vi "Build DashBoard Data.vi"(11 "Dashboard Enables":T3={"Analog Module 1"=[TRUE, TRUE, TRUE, TRUE, TRUE, TRUE, TRUE, TRUE], "Analog Module 2"=[FALSE, FALSE, FALSE, FALSE, FALSE, FALSE, FALSE, FALSE], "Digital Module 1"=TRUE, "Digital Module 2"=FALSE, "Solenoid Module"=TRUE}) -> ()   [LabVIEW 2012]
doc: "This VI builds data and sends it back to the dashboard PC program. By default it sends back the raw values for the first analog, digital, and solenoid module. Modify it to send back the data you want to view. Consider adding higher level data to the Dashboard Datatype.ctl and to this VI. Then update the Dashboard to display the data however you like.\n\nThis software is licensed. Open the labview\\readme\\WPI Robotics Library Open Source License.txt file for more information."
uses:
  DashboardEnable.ctl
  Dashboard Datatype.ctl
  <vilib>/Rock Robotics/WPI/DriverStation/WPI_DriverStationDigitalData.ctl
  Robot Global Data.vi
  <vilib>/Rock Robotics/SystemInterfaces/System/FPGA_SystemGet.vi
panel:
  out "Dashboard Data":T1
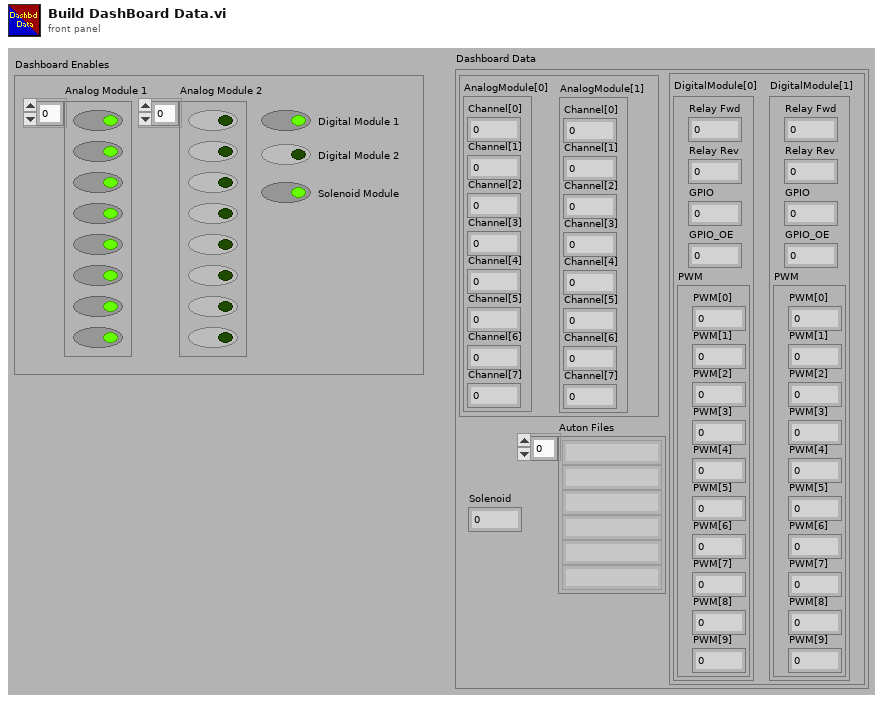
[diagram p1: front panel]
types:
  T1 = typedef "Dashboard Datatype.ctl" = cluster{cluster{"AnalogModule[0]":cluster{"Channel[0]":sgl, "Channel[1]":sgl, "Channel[2]":sgl, "Channel[3]":sgl, "Channel[4]":sgl, "Channel[5]":sgl, "Channel[6]":sgl, "Channel[7]":sgl}, "AnalogModule[1]":cluster{"Channel[0]":sgl, "Channel[1]":sgl, "Channel[2]":sgl, "Channel[3]":sgl, "Channel[4]":sgl, "Channel[5]":sgl, "Channel[6]":sgl, "Channel[7]":sgl}}, cluster{"DigitalModule[0]":T2, "DigitalModule[1]":T2}, "Solenoid":u8, "Auton Files":string[]}
  T2 = typedef "WPI_DriverStationDigitalData.ctl" = cluster{"Relay Fwd":u8, "Relay Rev":u8, "GPIO":u16, "GPIO_OE":u16, "PWM":cluster{"PWM[0]":u8, "PWM[1]":u8, "PWM[2]":u8, "PWM[3]":u8, "PWM[4]":u8, "PWM[5]":u8, "PWM[6]":u8, "PWM[7]":u8, "PWM[8]":u8, "PWM[9]":u8}}
  T3 = typedef "DashboardEnable.ctl" = cluster{"Analog Module 1":bool[], "Analog Module 2":bool[], "Digital Module 1":bool, "Digital Module 2":bool, "Solenoid Module":bool}
  T4 = cluster{"AnalogModule[0]":cluster{"Channel[0]":sgl, "Channel[1]":sgl, "Channel[2]":sgl, "Channel[3]":sgl, "Channel[4]":sgl, "Channel[5]":sgl, "Channel[6]":sgl, "Channel[7]":sgl}, "AnalogModule[1]":cluster{"Channel[0]":sgl, "Channel[1]":sgl, "Channel[2]":sgl, "Channel[3]":sgl, "Channel[4]":sgl, "Channel[5]":sgl, "Channel[6]":sgl, "Channel[7]":sgl}}
  T5 = cluster{"Channel[0]":sgl, "Channel[1]":sgl, "Channel[2]":sgl, "Channel[3]":sgl, "Channel[4]":sgl, "Channel[5]":sgl, "Channel[6]":sgl, "Channel[7]":sgl}[]
  T6 = cluster{"Channel[0]":sgl, "Channel[1]":sgl, "Channel[2]":sgl, "Channel[3]":sgl, "Channel[4]":sgl, "Channel[5]":sgl, "Channel[6]":sgl, "Channel[7]":sgl}
  T7 = cluster{"AnalogModule[0][0]":sgl, "AnalogModule[0][1]":sgl, "AnalogModule[0][2]":sgl, "AnalogModule[0][3]":sgl, "AnalogModule[0][4]":sgl, "AnalogModule[0][5]":sgl, "AnalogModule[0][6]":sgl, "AnalogModule[0][7]":sgl}
  T8 = cluster{"[0]":cluster{"Channel[0]":sgl, "Channel[1]":sgl, "Channel[2]":sgl, "Channel[3]":sgl, "Channel[4]":sgl, "Channel[5]":sgl, "Channel[6]":sgl, "Channel[7]":sgl}, "[1]":cluster{"Channel[0]":sgl, "Channel[1]":sgl, "Channel[2]":sgl, "Channel[3]":sgl, "Channel[4]":sgl, "Channel[5]":sgl, "Channel[6]":sgl, "Channel[7]":sgl}}
  T9 = cluster{"DigitalModule[0]":T2, "DigitalModule[1]":T2}
  T10 = typedef "FPGA_DIODevRef.ctl" = cluster{"DevStatus":errorcluster, "Module":T11}
  T11 = typedef "FPGA_TypedefDigitalModule.ctl" = enum16{"Digital Module 1", "Digital Module 2"}
  T12 = cluster{"[0]":u8, "[1]":u8, "[2]":u8, "[3]":u8, "[4]":u8, "[5]":u8, "[6]":u8, "[7]":u8, "[8]":u8, "[9]":u8}
  T13 = typedef "FPGA_SolenoidDevRef.ctl" = cluster{"DevStatus":errorcluster, "Module":T14}
  T14 = typedef "FPGA_TypedefSolenoidModule.ctl" = enum16{"Solenoid Module 1", "Solenoid Module 2"}
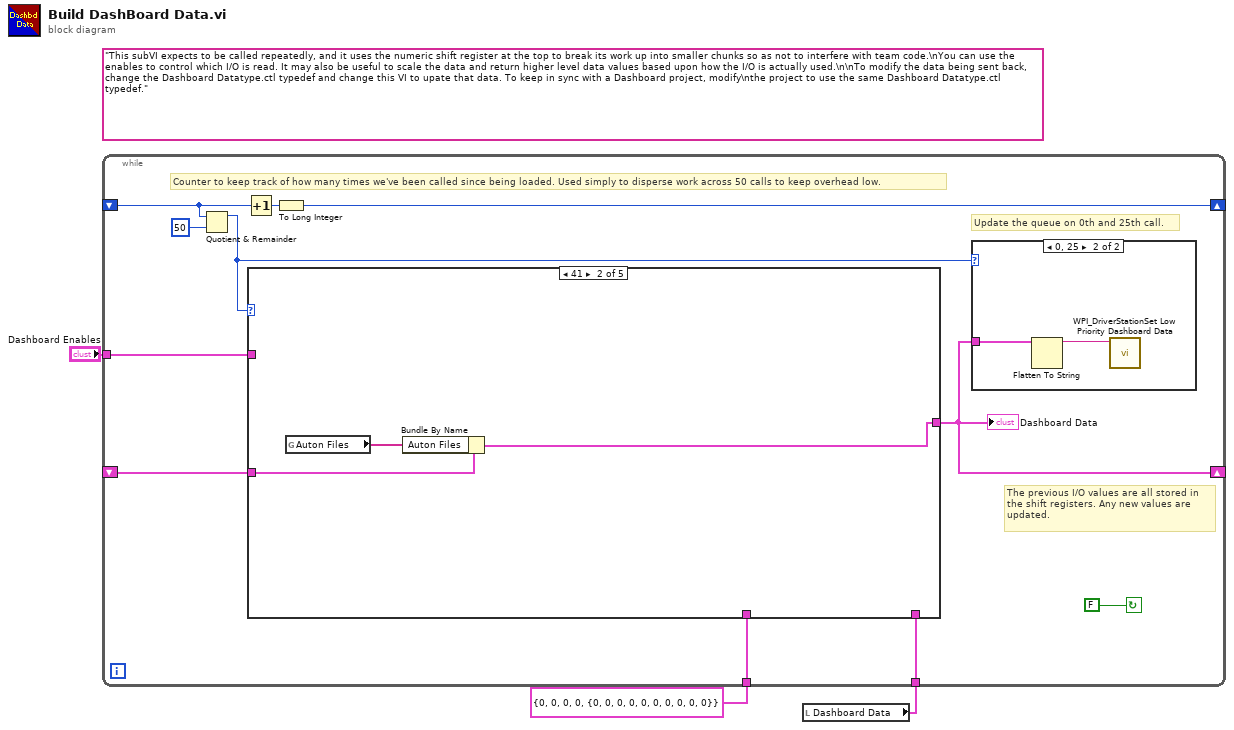
[diagram p0: block diagram]
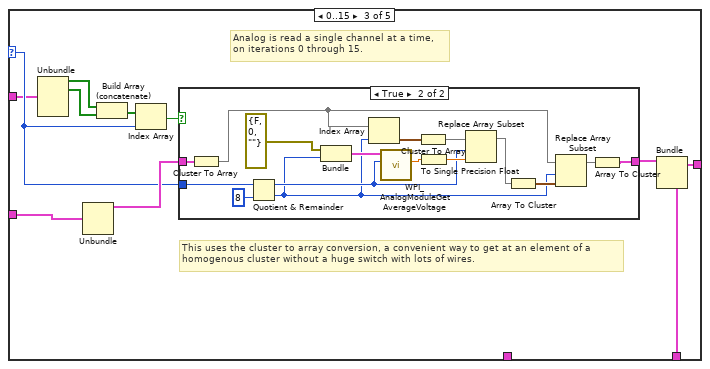
[diagram p4: hidden frame]
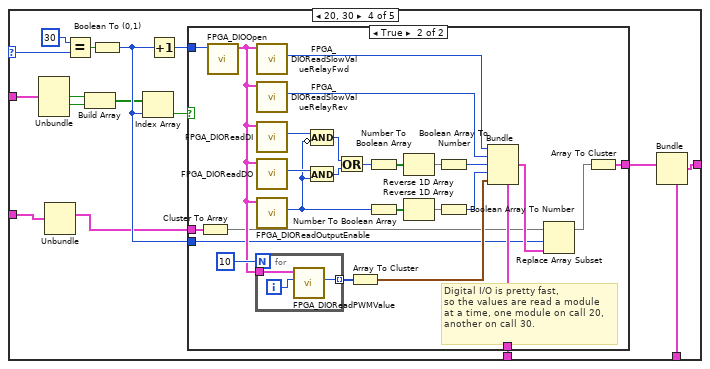
[diagram p6: hidden frame]
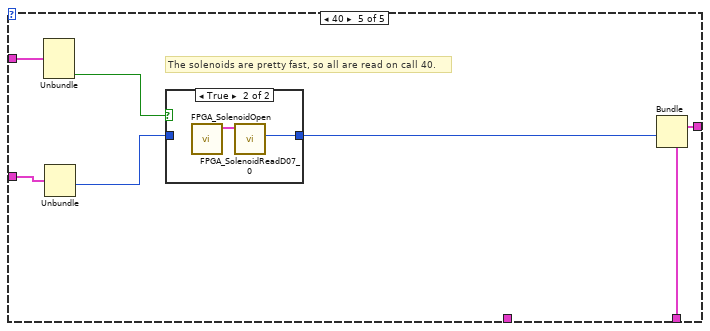
[diagram p8: hidden frame]
diagram:
  (unwired) "This subVI expects to be called repeatedly, and it uses the numeric shift register at the top to break its work up into smaller chunks so as not to interfere with team code.\nYou can use the enables to control which I/O is read. It may also be useful to scale the data and return higher level data values based upon how the I/O is actually used.\n\nTo modify the data being sent back, change the Dashboard Datatype.ctl typedef and change this VI to upate that data. To keep in sync with a Dashboard project, modify\nthe project to use the same Dashboard Datatype.ctl typedef."
  n1 = local read "Dashboard Data"() -> (w2:T1)
  n2 = while {
    shift-right: [w7] -> _
    shift-left: _ -> [w9]
    shift-right: [w4] -> _
    shift-left: _ -> [w12]
    tunnel: T2 {"Relay Fwd"=0, "Relay Rev"=0, "GPIO"=0, "GPIO_OE"=0, "PWM"={"PWM[0]"=0, "PWM[1]"=0, "PWM[2]"=0, "PWM[3]"=0, "PWM[4]"=0, "PWM[5]"=0, "PWM[6]"=0, "PWM[7]"=0, "PWM[8]"=0, "PWM[9]"=0}} ("DigitalModule[1]") -> [w11]
    tunnel: w2 -> [w6]
    tunnel: "Dashboard Enables" -> [w5]
    stop <- FALSE continue-if-true
    # "Counter to keep track of how many times we've been called since being loaded. Used simply to disperse work across 50 calls to keep overhead low."
    # "Update the queue on 0th and 25th call."
    # "The previous I/O values are all stored in\nthe shift registers. Any new values are\nupdated."
    n3 = Quotient & Remainder(x=w9, y=50) -> (x-y*floor(x/y)=w8:i32)  [unwired: 1 out]
    n4 = Increment(x=w9) -> (x+1=w14:i32)
    n5 = case shown="41" w8 {
      selector: w8 -> [_ _ w26 w58 _]
      tunnel: [w17 w19 w22 w49 w98] -> w4
      tunnel: w12 -> [w17 w20 w21 w51 w100]
      tunnel: w11 -> [_ _ _ w64 _]
      tunnel: w6 -> [_ _ w28 w50 w97]
      tunnel: w5 -> [_ _ w25 w56 w101]
      frame Default {
        # "Don't update any I/O"
      }
      frame 41 {
        n6 = global read "Robot Global Data.vi" "Auton Files"() -> (w18:string[])
        n7 = Bundle By Name(cluster=w20, "Auton Files"=w18) -> (w19:T1)
      }
      frame 0..15 {
        # "This uses the cluster to array conversion, a convenient way to get at an element of a\nhomogenous cluster without a huge switch with lots of wires."
        # "Analog is read a single channel at a time,\non iterations 0 through 15."
        n8 = Unbundle(w25) -> ("Analog Module 1"=w24:bool[], "Analog Module 2"=w23:bool[])  [unwired: 3 out]
        n9 = Unbundle(w21) -> (w27:T4)  [unwired: 3 out]
        n10 = Build Array (concatenate)(w24, w23) -> (w30:bool[])
        n11 = Index Array(array=w30, index=w26) -> (element=w31:bool)
        n12 = case shown="True" w31 {
          tunnel: w26 -> [_ w39]
          tunnel: [w32 w36] -> w29
          tunnel: w27 -> [w32 w35]
          frame False {
          }
          frame True {
            n13 = Cluster To Array(cluster=w35) -> (array=w34:T5)
            n14 = Quotient & Remainder(x=w39, y=8) -> (x-y*floor(x/y)=w38:i32, floor(x/y)=w33:i32)
            n15 = Bundle("DevStatus"=errorcluster {"status"=FALSE, "code"=0, "source"=""}, w33) -> (w47:cluster{"DevStatus":errorcluster, i32})  [unwired: 1 out]
            n16 = Index Array(array=w34, index=w33) -> (element=w41:T6)
            n17 = call <vilib>:"WPI_AnalogModuleGetAverageVoltage.vi"("Channel"=w38, "AnalogModuleDevStatus"=w47) -> ("Average Voltage"=w44:dbl)  [unwired: 1 in, 8 out]
            n18 = Cluster To Array(cluster=w41) -> (array=w40:sgl[])
            n19 = To Single Precision Float(number=w44) -> (single precision float=w43:sgl)
            n20 = Replace Array Subset(array=w40, new element=w43, index=w38) -> (w42:sgl[])
            n21 = Array To Cluster(array=w42) -> (cluster=w46:T7)
            n22 = Replace Array Subset(array=w34, new element=w46, index=w33) -> (w37:T5)
            n23 = Array To Cluster(array=w37) -> (cluster=w36:T8)
          }
        }
        n24 = Bundle(cluster=w28, w29) -> (w22:T1)  [unwired: 3 out]
      }
      frame 20, 30 {
        n25 = Unbundle(w56) -> ("Digital Module 1"=w55:bool, "Digital Module 2"=w54:bool)  [unwired: 3 out]
        n26 = Unbundle(w51) -> (w53:T9)  [unwired: 3 out]
        n27 = Equal?(x=30, y=w58) -> (x = y?=w62:bool)
        n28 = Build Array(w55, w54) -> (w57:bool[])
        n29 = Boolean To (0,1)(Boolean=w62) -> (0, 1=w60:i16)
        n30 = Index Array(array=w57, index=w60) -> (element=w59:bool)
        n31 = Increment(x=w60) -> (x+1=w61:i16)
        n32 = case shown="True" w59 {
          tunnel: w64 -> [_ w73]
          tunnel: [w65 w66] -> w52
          tunnel: w61 -> [_ w71]
          tunnel: w60 -> [_ w70]
          tunnel: w53 -> [w65 w69]
          frame False {
          }
          frame True {
            # "Digital I/O is pretty fast,\nso the values are read a module\nat a time, one module on call 20,\nanother on call 30."
            n33 = Cluster To Array(cluster=w69) -> (array=w68:T2[])
            n34 = call <vilib>:"FPGA_DIOOpen.vi"("Module (Module 1)"=w71) -> ("DIODeviceRef"=w89:T10)  [unwired: 1 in, 9 out]
            n35 = for {
              N: 10 -> [_]
              tunnel: w89 -> [w94]
              tunnel: [w92] -> w90 mode=indexing
              i -> [w93]
              n36 = call <vilib>:"FPGA_DIOReadPWMValue.vi"("PWMChannel"=w93, "DIODeviceRef In"=w94) -> ("PWMValue"=w92:u8)  [unwired: 1 in, 8 out]
            }
            n37 = call <vilib>:"FPGA_DIOReadSlowValueRelayFwd.vi"("DIODeviceRef In"=w89) -> ("Relay Forward"=w82:u8)  [unwired: 1 in, 9 out]
            n38 = call <vilib>:"FPGA_DIOReadSlowValueRelayRev.vi"("DIODeviceRef In"=w89) -> ("Relay Reverse"=w83:u8)  [unwired: 1 in, 9 out]
            n39 = call <vilib>:"FPGA_DIOReadDI.vi"("DIODeviceRef In"=w89) -> ("DI"=w87:u16)  [unwired: 1 in, 9 out]
            n40 = call <vilib>:"FPGA_DIOReadDO.vi"("DIODeviceRef In"=w89) -> ("DO"=w86:u16)  [unwired: 1 in, 9 out]
            n41 = call <vilib>:"FPGA_DIOReadOutputEnable.vi"("DIODeviceRef In"=w89) -> ("OutputEnable"=w77:u16)  [unwired: 1 in, 9 out]
            n42 = And(x=w86, y=w77) -> (x .and. y?=w85:u16)
            n43 = Compound Arithmetic op=AND(w87, invert w77) -> (w84:u16)
            n44 = Or(x=w84, y=w85) -> (x .or. y?=w75:u16)
            n45 = Array To Cluster(array=w90) -> (cluster=w88:T12)
            n46 = Number To Boolean Array(number=w75) -> (Boolean array=w80:bool[])
            n47 = Number To Boolean Array(number=w77) -> (Boolean array=w79:bool[])
            n48 = Reverse 1D Array(array=w80) -> (reversed array=w81:bool[])
            n49 = Reverse 1D Array(array=w79) -> (reversed array=w78:bool[])
            n50 = Boolean Array To Number(Boolean array=w81) -> (number=w74:u32)
            n51 = Boolean Array To Number(Boolean array=w78) -> (number=w76:u32)
            n52 = Bundle(cluster=w73, "Relay Fwd"=w82, "Relay Rev"=w83, "GPIO"=w74, "GPIO_OE"=w76, "PWM"=w88) -> (w72:T2)
            n53 = Replace Array Subset(array=w68, new element=w72, index=w70) -> (w67:T2[])
            n54 = Array To Cluster(array=w67) -> (cluster=w66:cluster{"[0]":T2, "[1]":T2})
          }
        }
        n55 = Bundle(cluster=w50, w52) -> (w49:T1)  [unwired: 3 out]
      }
      frame 40 {
        # "The solenoids are pretty fast, so all are read on call 40."
        n56 = Unbundle(w101) -> ("Solenoid Module"=w95:bool)  [unwired: 4 out]
        n57 = Unbundle(w100) -> ("Solenoid"=w99:u8)  [unwired: 3 out]
        n58 = case shown="True" w95 {
          tunnel: [w102 w103] -> w96
          tunnel: w99 -> [w102 _]
          frame False {
          }
          frame True {
            n59 = call <vilib>:"FPGA_SolenoidOpen.vi"() -> ("SolenoidDevRef"=w104:T13)  [unwired: 2 in, 9 out]
            n60 = call <vilib>:"FPGA_SolenoidReadD07_0.vi"("SolenoidDevRef"=w104) -> ("DO7:0"=w103:u8)  [unwired: 1 in, 9 out]
          }
        }
        n61 = Bundle(cluster=w97, "Solenoid"=w96) -> (w98:T1)  [unwired: 3 out]
      }
    }
    "Dashboard Data" <- w4
    n62 = To Long Integer(number=w14) -> (32bit integer=w7:i32)
    n63 = case shown="0, 25" w8 {
      tunnel: w4 -> [_ w16]
      frame Default {
      }
      frame 0, 25 {
        n64 = Flatten To String(anything=w16) -> (data string=w15:string)  [unwired: 1 in, 4 out]
        n65 = call <vilib>:"WPI_DriverStationSet Low Priority Dashboard Data.vi"("User Data"=w15) -> ()  [unwired: 1 in, 10 out]
      }
    }
  }
